vi "ShooterLights.vi"   [LabVIEW 2011]
uses:
  <vilib>/Rock Robotics/WPI/Relay/WPI_RelayValue.ctl
  System Set Points and States.vi
types:
  T1 = typedef "WPI_RelayDevRef.ctl" = cluster{"DevStatus":errorcluster, "Relay Channel":T2, "Digital Module":T3, "Relay Direction":T4}
  T2 = typedef "FPGA_DIORelayChannel.ctl" = enum8{"Relay 1", "Relay 2", "Relay 3", "Relay 4", "Relay 5", "Relay 6", "Relay 7", "Relay 8", "Invalid"}
  T3 = typedef "FPGA_TypedefDigitalModule.ctl" = enum16{"Digital Module 1", "Digital Module 2"}
  T4 = typedef "WPI_RelayDirection.ctl" = enum16{"Both directions", "Forward only", "Reverse only"}
  T5 = typedef "WPI_RelayValue.ctl" = enum16{"Off", "On", "Forward", "Reverse"}
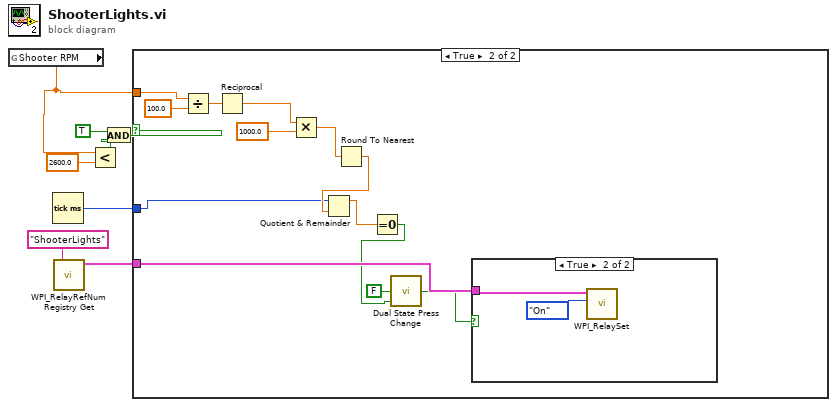
[diagram p0: block diagram]
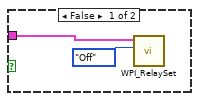
[diagram p3: hidden frame]
diagram:
  n1 = global read "System Set Points and States.vi" "Shooter RPM"() -> (w8:dbl)
  n2 = Tick Count (ms)() -> (millisecond timer value=w2:u32)
  n3 = call <vilib>:"WPI_RelayRefNum Registry Get.vi"("refnum name"="ShooterLights") -> ("RelayDevRef"=w3:T1)  [unwired: 9 in, 1 out]
  n4 = Less?(x=w8, y=2600.0) -> (x < y?=w5:bool)
  n5 = And(x=TRUE, y=w5) -> (x .and. y?=w6:bool)
  n6 = case shown="True" w6 {
    tunnel: w8 -> [_ w15]
    tunnel: w3 -> [_ w19]
    tunnel: w2 -> [_ w11]
    frame False {
    }
    frame True {
      n7 = Divide(x=w15, y=100.0) -> (x/y=w14:dbl)
      n8 = Reciprocal(x=w14) -> (1/x=w13:dbl)
      n9 = Multiply(x=w13, y=1000.0) -> (x*y=w16:dbl)
      n10 = Round To Nearest(number=w16) -> (nearest integer value=w12:dbl)
      n11 = Quotient & Remainder(x=w11, y=w12) -> (x-y*floor(x/y)=w10:dbl)  [unwired: 1 out]
      n12 = Equal To 0?(x=w10) -> (x = 0?=w9:bool)
      n13 = call "Dual State Press Change.vi"("Enable/Disable"=w9, "Initial"=FALSE) -> ("Enabled"=w18:bool)  [unwired: 1 in]
      n14 = case shown="True" w18 {
        tunnel: w19 -> [w23 w25]
        frame False {
          n15 = call <vilib>:"WPI_RelaySet.vi"("RelayValue"=WPI_RelayValue."Off", "RelayDevRef"=w23) -> ()  [unwired: 8 in, 2 out]
        }
        frame True {
          n16 = call <vilib>:"WPI_RelaySet.vi"("RelayValue"=WPI_RelayValue."On", "RelayDevRef"=w25) -> ()  [unwired: 8 in, 2 out]
        }
      }
    }
  }
